vi "Husky Loop.vi"() -> ()   [LabVIEW 2011]
uses:
  <vilib>/Platform/TimedLoop/XDataNode/timing_clust.ctl
  <vilib>/Platform/TimedLoop/XDataNode/nitl_modes.ctl
  <vilib>/Platform/TimedLoop/XDataNode/wakeup.ctl
  <vilib>/Platform/TimedLoop/XDataNode/XDataNode.xnode
  clearpath_interface.lvlib
  <vilib>/Platform/TimedLoop/XDataNode/XDNodeRunTimeDep.lvlib
panel:
  in  "VISA resource name":refnum<visa-resource-name>
  in  "Debug":bool
  out "Charge":dbl(slide) scale=0.0..100.0
  out "Left Speed (m/s)":dbl
  out "Right Speed (m/s)":dbl
  out "Capacity":i16
  out "Flags":u8 format="%b"
  out "Flags 2":u8 format="%x"
  out "Telemetry":T1={"Voltage"={0.0, 0.0, 0.0}, "Encoder Speed"={0, 0}, "Temps"={"IC Temp (C)"=0, "Ch1 Temp (C)"=0, "Ch2 Temp (C)"=0}, "Current"={0.0, 0.0, 0.0, 4.6238981750249924e+36}} {"Current" scale=0.0..16.0; "Temps"."IC Temp (C)" scale=0.0..150.0; "Temps"."Ch1 Temp (C)" scale=0.0..150.0; "Temps"."Ch2 Temp (C)" scale=0.0..150.0; "Encoder Speed" scale=-100.0..100.0; "Voltage" scale=8.0..14.0}
  in  "End Loop":bool
  in  "stop?":bool
  in  "Max Speed (m/s)":dbl
  in  "Max Accel (m/s/s)":dbl
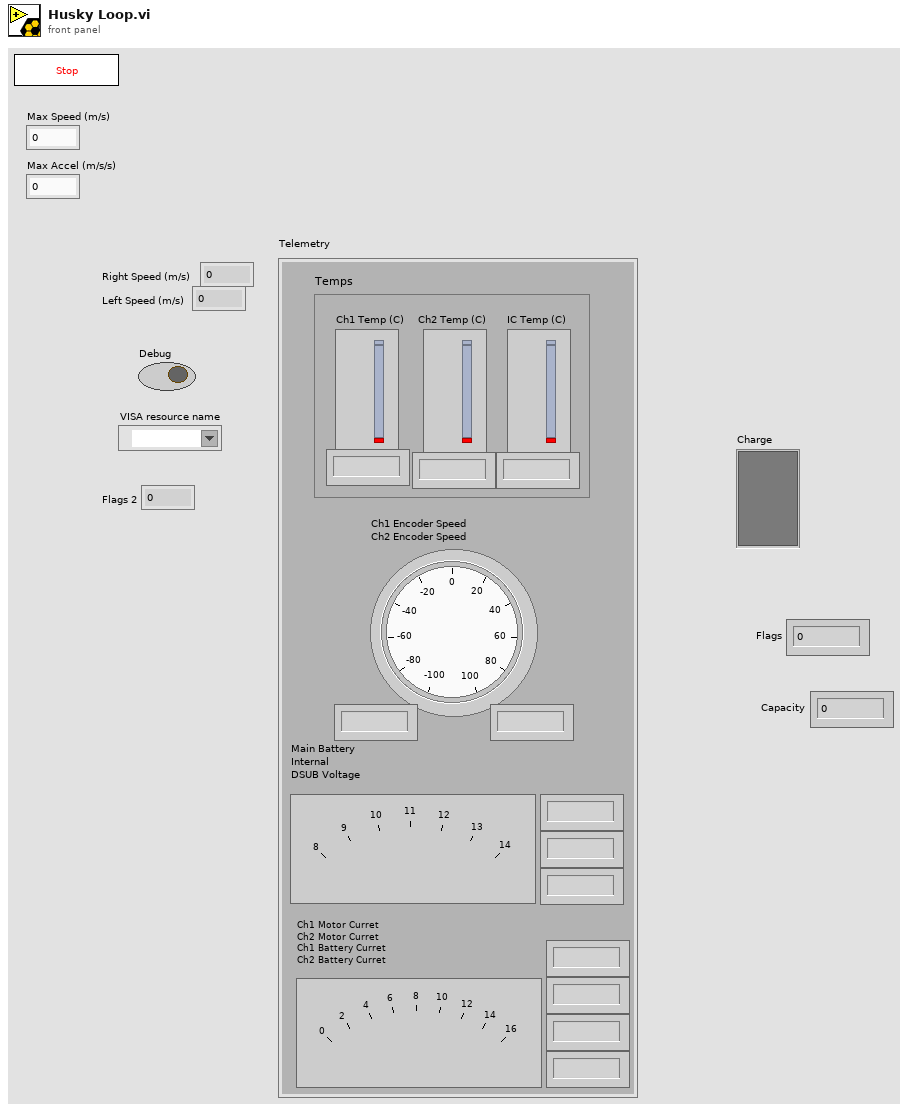
[diagram p1: front panel]
types:
  T1 = cluster{"Voltage":cluster{sgl, sgl, sgl}, "Encoder Speed":cluster{i32, i32}, "Temps":cluster{"IC Temp (C)":i32, "Ch1 Temp (C)":i32, "Ch2 Temp (C)":i32}, "Current":cluster{dbl, dbl, dbl, dbl}}
  T2 = cluster{"Xmit Queue":refnum<queue>, "Data Queue":refnum<queue>, "VISA resource name out":refnum<visa-resource-name>, "error out":errorcluster, "Message Data Cluster":cluster{"\nChar Idx":u8, "Num. Char Rem":u8, "Write Index":u8, "Read Index":u8, "Message Data Buffer":u8[][]}}
  T3 = typedef "XDNodeRunTimeDep.lvlib/timing_clust.ctl" = cluster{"Expected End [f-1]":u64, "Actual End [f-1]":u64, "Finished Late? [f-1]":bool, "Expected End [i-1]":u64, "Actual End [i-1]":u64, "Finished Late? [i-1]":bool, "Expected Start [i]":u64, "Actual Start [i]":u64, "Expected Start [f]":u64, "Actual Start [f]":u64, "Source Name":string, "Structure Name":string, "Period":i64, "Deadline":i64, "Offset":i64, "Start":i64, "Priority":i32, "Timeout":i32, "Mode":T4, "Wakeup Reason":T5, "Error":errorcluster, "Source Type":string, "Secondary Source Type":string, "Global End Time":u64, "Global Start Time":u64, "Frame Duration":u64, "Iteration Duration":u64, "Assigned CPU":i32, "I/O Scan Engine Mode":u32}
  T4 = typedef "XDNodeRunTimeDep.lvlib/nitl_modes.ctl" = enum32{"No Change", "Process missed periods, maintain original phase", "Discard missed periods, maintain original phase", "Process missed periods, ignore original phase", "Discard missed periods, ignore original phase"}
  T5 = typedef "XDNodeRunTimeDep.lvlib/wakeup.ctl" = enum32{"Normal", "Aborted", "Asynchronous wakeup", "Timing source error", "Timed loop error", "Timeout"}
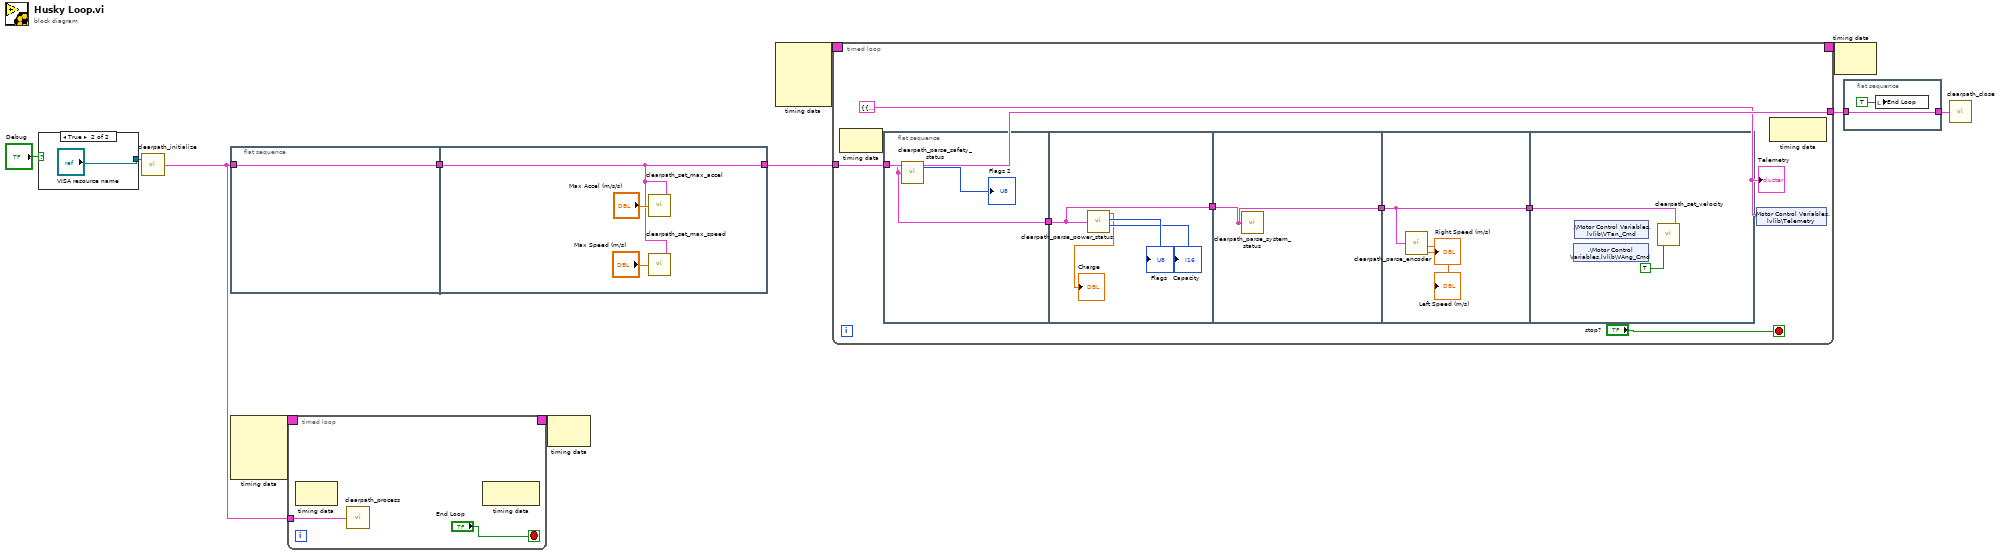
[diagram p0: block diagram]
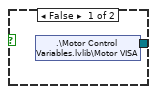
[diagram p2: hidden frame]
diagram:
  n1 = case shown="True" "Debug" {
    tunnel: [w12 "VISA resource name"] -> w9
    frame False {
      n2 = shared-variable ".\\Motor Control Variables.lvlib\\Motor VISA"() -> (w12:refnum<visa-resource-name>)  [unwired: 1 in, 1 out]
    }
    frame True {
    }
  }
  n3 = call "clearpath_initialize.vi"("VISA resource name"=w9) -> ("ClearpathComm"=w8:T2)  [unwired: 1 in]
  n4 = flat-sequence {
    tunnel: w8 -> [w14]
    tunnel: [w14] -> w7
    tunnel: w7 -> [w15]
    tunnel: [w15] -> w4
    frame #0 {
    }
    frame #1 {
      n5 = call "clearpath_set_max_accel.vi"("ClearpathComm"=w15, "Max Accel"="Max Accel (m/s/s)") -> ()
      n6 = call "clearpath_set_max_speed.vi"("ClearpathComm"=w15, "Max Speed"="Max Speed (m/s)") -> ()
    }
  }
  n7 = node-c288() -> (w11:T3)  [unwired: 4 in]
  n8 = timed-loop {
    timing: w11 -> [_]
    timing-out: [_] -> w10
    tunnel: w8 -> [w19]
    stop <- "End Loop" stop-if-true
    n9 = node-c288() -> ()  [unwired: 1 in, 1 out]
    n10 = call "clearpath_process.vi"("ClearpathComm"=w19) -> ()
    n11 = node-c288() -> ()  [unwired: 1 in, 1 out]
  }
  n12 = node-c288(w10) -> ()  [unwired: 1 out]
  n13 = node-c288() -> (w6:T3)  [unwired: 4 in]
  n14 = timed-loop {
    timing: w6 -> [_]
    timing-out: [_] -> w5
    tunnel: w4 -> [w27]
    tunnel: [w27] -> w2
    stop <- "stop?" stop-if-true
    w22 = T1 {"Voltage"={0.0, 0.0, 0.0}, "Encoder Speed"={0, 0}, "Temps"={"IC Temp (C)"=0, "Ch1 Temp (C)"=0, "Ch2 Temp (C)"=0}, "Current"={0.0, 0.0, 0.0, 0.0}} ("Telemetry")
    n15 = node-c288() -> ()  [unwired: 1 in, 1 out]
    n16 = flat-sequence {
      tunnel: w27 -> [w29]
      tunnel: [w29] -> w26
      tunnel: w26 -> [w32]
      tunnel: [w32] -> w25
      tunnel: [w35] -> w24
      tunnel: w25 -> [w35]
      tunnel: w24 -> [w38]
      tunnel: [w38] -> w23
      tunnel: w23 -> [w40]
      frame #0 {
        n17 = call "clearpath_parse_safety_status.vi"("ClearpathComm"=w29) -> ("Flags"=→"Flags 2":u8)  [unwired: 1 out]
      }
      frame #1 {
        n18 = call "clearpath_parse_power_status.vi"("ClearpathComm"=w32) -> ("Capacity"=→"Capacity":i16, "Flags"=→"Flags":u8, "Charge"=→"Charge":dbl)  [unwired: 1 out]
      }
      frame #2 {
        n19 = call "clearpath_parse_system_status.vi"("ClearpathComm"=w35) -> ()  [unwired: 6 out]
      }
      frame #3 {
        n20 = call "clearpath_parse_encoder.vi"("ClearpathComm"=w38) -> ("Left Speed (m/s)"=→"Left Speed (m/s)":dbl, "Right Speed (m/s)"=→"Right Speed (m/s)":dbl)  [unwired: 3 out]
      }
      frame #4 {
        n21 = shared-variable ".\\Motor Control Variables.lvlib\\VAng_Cmd"() -> ()  [unwired: 1 in, 2 out]
        n22 = shared-variable ".\\Motor Control Variables.lvlib\\VTan_Cmd"() -> ()  [unwired: 1 in, 2 out]
        n23 = call "clearpath_set_velocity.vi"("ClearpathComm"=w40, "Zero Speeds"=TRUE) -> ()  [unwired: 2 in]
      }
    }
    n24 = shared-variable ".\\Motor Control Variables.lvlib\\Telemetry"(w22) -> ()  [unwired: 1 in, 1 out]
    n25 = node-c288() -> ()  [unwired: 1 in, 1 out]
    "Telemetry" <- w22
  }
  n26 = node-c288(w5) -> ()  [unwired: 1 out]
  n27 = flat-sequence {
    tunnel: [w43] -> w3
    tunnel: w2 -> [w43]
    frame #0 {
      n28 = local write "End Loop"(TRUE ("End Loop")) -> ()
    }
  }
  n29 = call "clearpath_close.vi"("ClearpathComm"=w3) -> ()
